vi "Configure NofBins.vi"(8 "error in (no error)":errorcluster, 10 "NofBins":i32, 11 "CS++MCS in":refnum<class "CS++MCS.lvclass">) -> (0 "error out":errorcluster, 3 "CS++MCS out":refnum<class "CS++MCS.lvclass">)   [LabVIEW 2015, in "CS++MCS.lvlib" / "CS++MCS.lvclass"]
doc: "This VI configures the Number of Bins in the recorded spectrum."
uses:
  CS++MCS.lvclass
  CSPP_Core/Classes/CS++ProcessVariables/ProcessVariable/PV.lvclass
  PV-Enum.ctl
  CSPP_Core/Classes/CS++ProcessVariables/ProcessVariable/PV.lvclass/PV.ctl
  CS++MCS.lvclass/CS++MCS.ctl
  CSPP_Core/Classes/CS++ProcessVariables/ProcessVariable/Write Data.vi
  CSPP_Core/Classes/CS++ProcessVariables/ProcessVariable/Write Timestamp.vi
  CSPP_Core/Classes/CS++ProcessVariables/ProcessVariable/Write Quality.vi
  CSPP_Core/Classes/CS++ProcessVariables/ProcessVariable/Write status.vi
  CSPP_Core/Classes/CS++ProcessVariables/PVConnection/PVConnection.lvclass
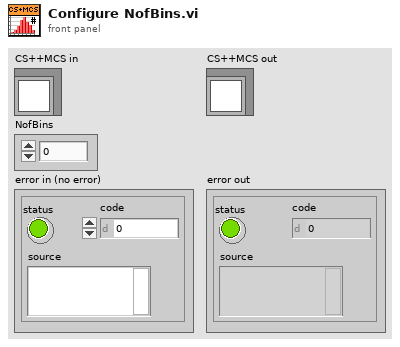
[diagram p1: front panel]
types:
  T1 = typedef "CS++MCS.lvlib/CS++MCS.lvclass/PV-Enum.ctl" = enum16{"Counts/I32", "TotalCounts/I32", "Status/I8", "BinWidth/Dbl", "NofBins/I32", "NofRecords /I32", "DiscLvl/Dbl", "TrigLvl/Dbl", "DiscSlope/U16", "TrigSlope/U16", "ActWaveform/AWfm|0:1"}
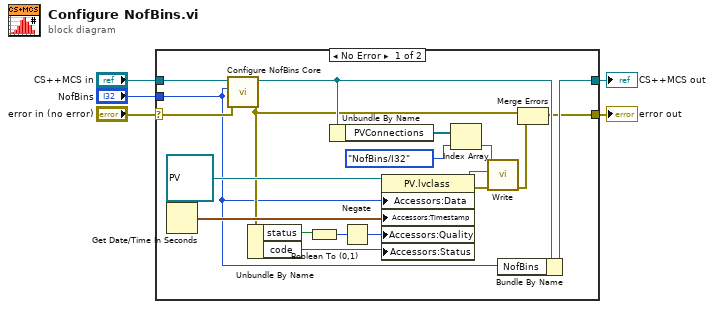
[diagram p0: block diagram]
diagram:
  n1 = case shown="No Error" "error in (no error)" {
    selector: "error in (no error)" -> [w23 w26]
    tunnel: [w9 w26] -> w4
    tunnel: [w11 w25] -> w2
    tunnel: "CS++MCS in" -> [w24 w25]
    tunnel: "NofBins" -> [w7 _]
    frame No Error {
      n2 = Get Date/Time In Seconds() -> (seconds since 1Jan1904=w14:timestamp)
      n3 = call-dynamic "Configure NofBins Core.vi"("error in (no error)"=w23, "NofBins"=w7, "CS++MCS in"=w24) -> ("error out"=w10:errorcluster, "CS++MCS out"=w12:refnum<class "CS++MCS.lvclass">)  [unwired: 7 in]
      n4 = Unbundle By Name(w10) -> ("status"=w18:bool, "code"=w20:i32)
      n5 = Boolean To (0,1)(Boolean=w18) -> (0, 1=w19:i16)
      n6 = Unbundle By Name(w12) -> ("PVConnections"=w22:refnum<class "PVConnection.lvclass">[])
      n7 = Negate(x=w19) -> (-x=w21:i16)
      n8 = property class="PV.lvclass"(reference=refnum<class "PV.lvclass"> refnum ("PV"), "Accessors:Data"=w7, "Accessors:Timestamp"=w14, "Accessors:Quality"=w21, "Accessors:Status"=w20) -> (reference out=w17:refnum<class "PV.lvclass">, error out=w16:errorcluster)  [unwired: 1 in]
      n9 = Index Array(array=w22, index=PV-Enum."NofBins/I32" ("PV-Enum")) -> (element=w13:refnum<class "PVConnection.lvclass">)
      n10 = call "Write.vi"("error in (no error)"=w16, "PV"=w17, "PVConnection in"=w13) -> ("error out"=w8:errorcluster)  [unwired: 7 in, 1 out]
      n11 = Bundle By Name(cluster=w12, "NofBins"=w7) -> (w11:refnum<class "CS++MCS.lvclass">)
      n12 = Merge Errors(w10, w8) -> (w9:errorcluster)
    }
    frame Error {
    }
  }
  "error out" <- w4
  "CS++MCS out" <- w2
